vi "init.vi"(8 "error in (no error)":errorcluster, 10 "Init Data":variant, 11 "MKS in":refnum<class "MKS.lvclass">) -> (0 "error out":errorcluster, 2 "Channel List":refnum<class "HK Item.lvclass">[](array[class]), 3 "MKS out":refnum<class "MKS.lvclass">)   [LabVIEW 2022 SP3, in "MKS.lvclass"]
uses:
  MKS.lvclass
  hk-channel-class/hk-channel-class/HK Item/HK Item.lvclass
  hk-channel-class/hk-channel-class/HK Item/HK Channel Units and Setup.ctl
  hk-channel-class/hk-channel-class/HK Item/HK Channel enum Data Type.ctl
  MKS.lvclass/MKS.ctl
  Pressure Monitor.lvclass
  <instrlib>/MKS 972B/MKS 972B.lvlib
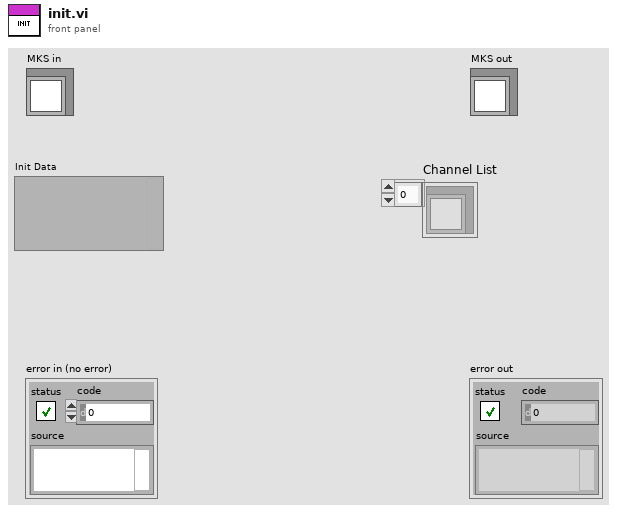
[diagram p1: front panel]
types:
  T1 = typedef "HK Item.lvclass/HK Channel Units and Setup.ctl" = cluster{"Unit Type":string, "Units":string, "Configuration":string, "Digits":i32, "Data Type":T2, "Exponential?":bool, "Source":string}
  T2 = typedef "HK Item.lvclass/HK Channel enum Data Type.ctl" = enum16{"Floating Point", "Integer", "Enum", "String", "Waveform", "File"}
  T3 = typedef "MKS.lvclass/MKS Settings.ctl" = cluster{"Serial Configuration":cluster{"Baud Rate":u32, "Parity":u16, "Data Bits":u16, "Stop Bits":u16, "Flow Control":u16}, "VISA resource name":refnum<visa-resource-name>, "Unit address":T4}
  T4 = typedef "MKS 972B.lvlib/Unit address.ctl" = u32
  T5 = cluster{"Baud Rate":u32, "Parity":u16, "Data Bits":u16, "Stop Bits":u16, "Flow Control":u16}
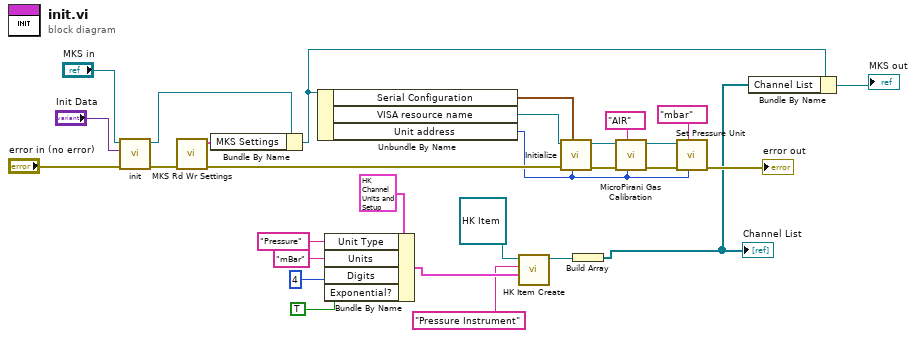
[diagram p0: block diagram]
diagram:
  n1 = call-parent "init.vi"("error in (no error)"="error in (no error)", "Init Data"="Init Data", "Pressure Monitor in"="MKS in") -> ("error out"=w8:errorcluster, "Pressure Monitor out"=w6:refnum<class "MKS.lvclass">)  [unwired: 6 in, 1 out]
  n2 = call "MKS Rd Wr Settings.vi"("error in (no error)"=w8) -> ("error out"=w5:errorcluster, "MKS Settings"=w7:T3)  [unwired: 9 in]
  n3 = Bundle By Name(cluster=w6, "MKS Settings"=w7) -> (w3:refnum<class "MKS.lvclass">)
  n4 = Unbundle By Name(w3) -> ("Serial Configuration"=w24:T5, "VISA resource name"=w23:refnum<visa-resource-name>, "Unit address"=w4:T4)
  n5 = Bundle By Name(cluster=T1 {"Unit Type"="", "Units"="", "Configuration"="", "Digits"=3, "Data Type"=enum."Floating Point", "Exponential?"=FALSE, "Source"=""} ("Channel Setup"), "Unit Type"="Pressure", "Units"="mBar", "Digits"=4, "Exponential?"=TRUE) -> (w12:T1)
  n6 = call-dynamic "HK Item Create.vi"("Channel Setup"=w12, "Name"="Pressure Instrument", "HK Item in"=refnum<class "HK Item.lvclass"> refnum) -> ("HK Item out"=w9:refnum<class "HK Item.lvclass">)  [unwired: 7 in, 1 out]
  n7 = call <instrlib>:"Initialize.vi"("Unit address to query ID (001-254)"=w4, "Serial Configuration"=w24, "error in (no error)"=w5, "VISA resource name"=w23) -> ("error out"=w26:errorcluster, "VISA resource name out"=w25:refnum<visa-resource-name>)  [unwired: 6 in]
  n8 = Build Array(w9) -> (w2:refnum<class "HK Item.lvclass">[])
  "Channel List" <- w2
  n9 = call <instrlib>:"MicroPirani Gas Calibration.vi"("Unit address (001-253)"=w4, "Calibration gas type"="AIR", "error in (no error)"=w26, "VISA resource name"=w25) -> ("error out"=w20:errorcluster, "VISA resource name out"=w21:refnum<visa-resource-name>)  [unwired: 6 in]
  n10 = call <instrlib>:"Set Pressure Unit.vi"("Unit address (001-253)"=w4, "Pressure unit"="mbar", "error in (no error)"=w20, "VISA resource name"=w21) -> ("error out"=→"error out":errorcluster)  [unwired: 6 in, 1 out]
  n11 = Bundle By Name(cluster=w3, "Channel List"=w2) -> (→"MKS out":refnum<class "MKS.lvclass">)
